vi "Self Execution.vi"(6 "Any Data In":variant, 7 "Any Data 2 In":variant, 8 "error in (no error)":errorcluster, 9 "Self Addressed Task In":refnum<class "Self Addressed Task.lvclass">, 10 "Message In":refnum<class "Message.lvclass">, 11 "Actor In":refnum<class "System Actor.lvclass">) -> (0 "error out":errorcluster, 1 "Self Addressed Task Out":refnum<class "Self Addressed Task.lvclass">, 2 "Message Out":refnum<class "Message.lvclass">, 3 "Actor Out":refnum<class "System Actor.lvclass">, 4 "Any Data Out":variant, 5 "Any Data 2 Out":variant)   [LabVIEW 2024, in "Self Addressed Task.lvclass"]
uses:
  Self Addressed Task.lvclass
  Actor/System Actor/System Actor.lvclass
  Message/Message.lvclass
  C:/Users/iio/Desktop/Bussiness/Tricorn Re/Madelbrot 4.0/General Library/Ancestor Class/Task/Task Ancestor/Task Ancestor.lvclass
  Task Ancestor/Task Ancestor.lvclass/Task Ancestor.ctl
  Self Addressed Task.lvclass/Self Addressed Task.ctl
  Task Ancestor/Public Data/Write Any Data.vi
  Public Data/Read Return Address.vi
  Task Ancestor/Task Ancestor.lvclass
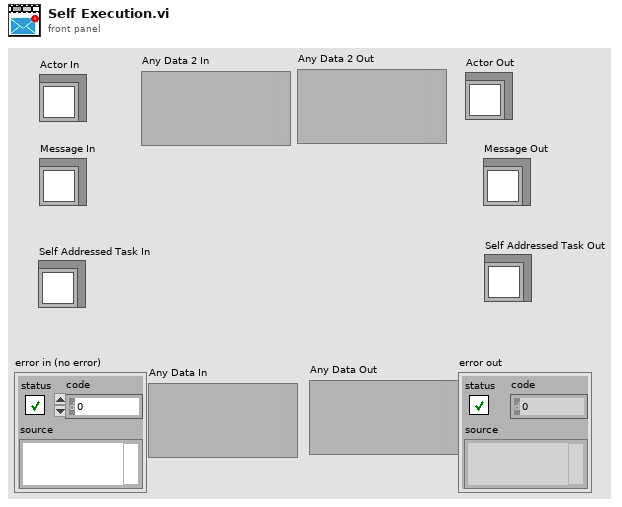
[diagram p1: front panel]
types:
  T1 = typedef "Return Address.ctl" = refnum<queue>
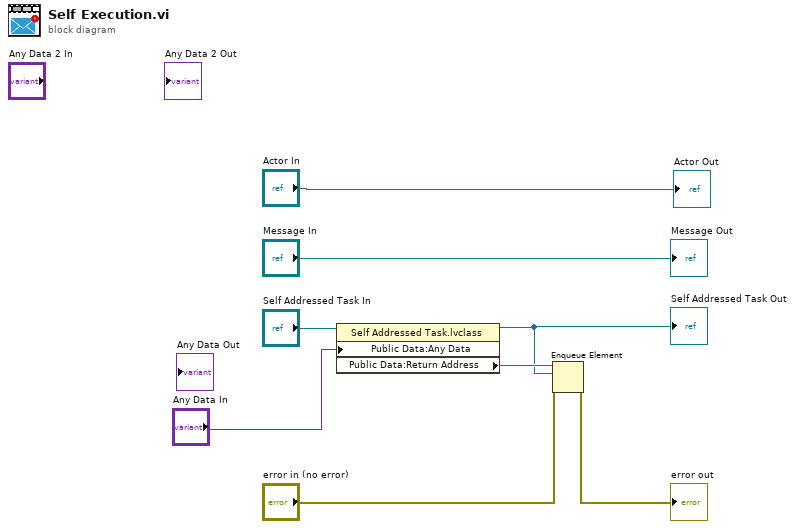
[diagram p0: block diagram]
diagram:
  n1 = property class="Self Addressed Task.lvclass"(reference="Self Addressed Task In", "Public Data:Any Data"="Any Data In") -> (reference out=w5:refnum<class "Self Addressed Task.lvclass">, "Public Data:Return Address"=w6:T1)  [unwired: 1 in, 1 out]
  "Self Addressed Task Out" <- w5
  n2 = Enqueue Element(queue=w6, element=w5, error in (no error)="error in (no error)") -> (error out=→"error out":errorcluster)  [unwired: 1 in, 2 out]
  "Message Out" <- "Message In"
  "Actor Out" <- "Actor In"
